vi "RFmx_An_IMD_Disp.vi"(6 "Target_Pwr(dBm)":dbl=1000000.0 format="%#_6p", 8 "Int_Bandwidth(Hz)":dbl=1000000.0 format="%#_6p", 9 "Signal_Bandwidth(Hz)":dbl=20000000.0 format="%#_6p", 10 "Tone_Spacing(Hz)":dbl=3000000.0 format="%#_6p", 11 "IMD_Spectrum_in":cluster{"x0":dbl, "dx":dbl, "y":sgl[]}={"x0"=989999984.4503028, "dx"=999.4019138756557, "y"=array[20012 elements]}) -> (2 "PeakPwrs_Data":sgl[](array[numeric])=[750000.0, -20.734814, 53.66733, 3.5194657] format="%#_6p", 3 "IMD_Spectrum_Out":cluster{"x0":dbl, "dx":dbl, "y":sgl[]}[](array[cluster])=[{"x0"=989999984.4503028, "dx"=999.4019138756557, "y"=array[20012 elements]}, {"x0"=989999984.4503028, "dx"=999.4019138756557, "y"=array[20012 elements]}])   [LabVIEW 2014]
panel:
  out "IMD_Spectrum":cluster{"x0":dbl, "dx":dbl, "y":sgl[]}[](graph)
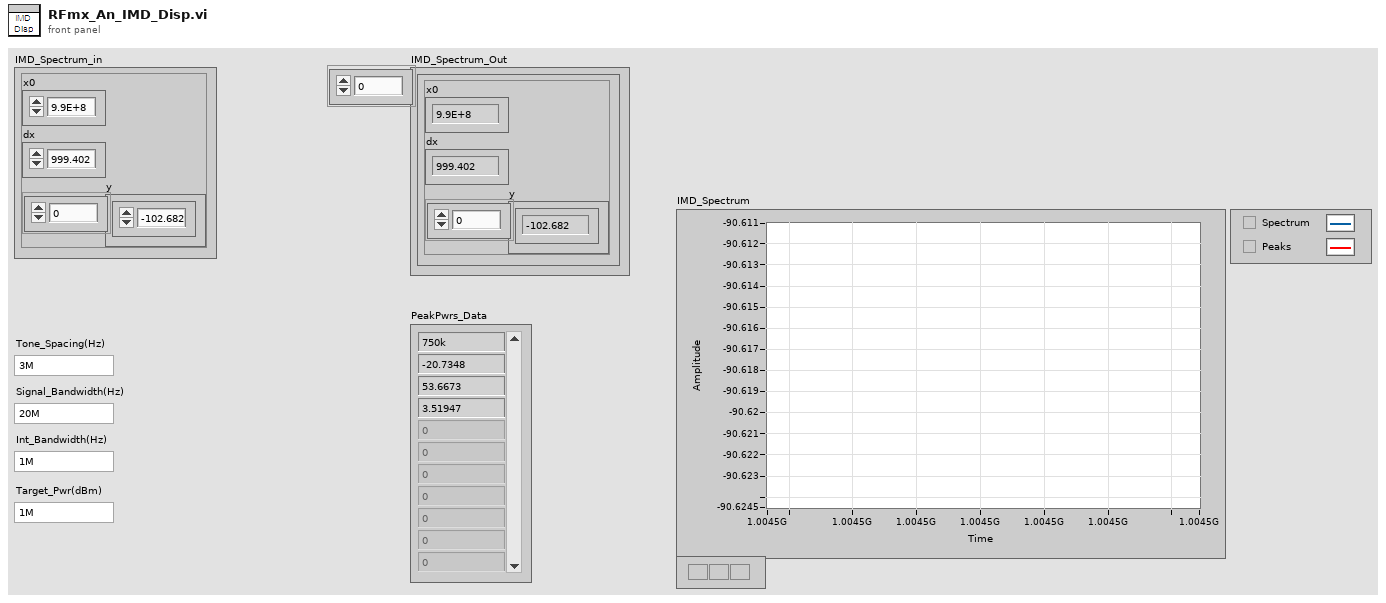
[diagram p1: front panel]
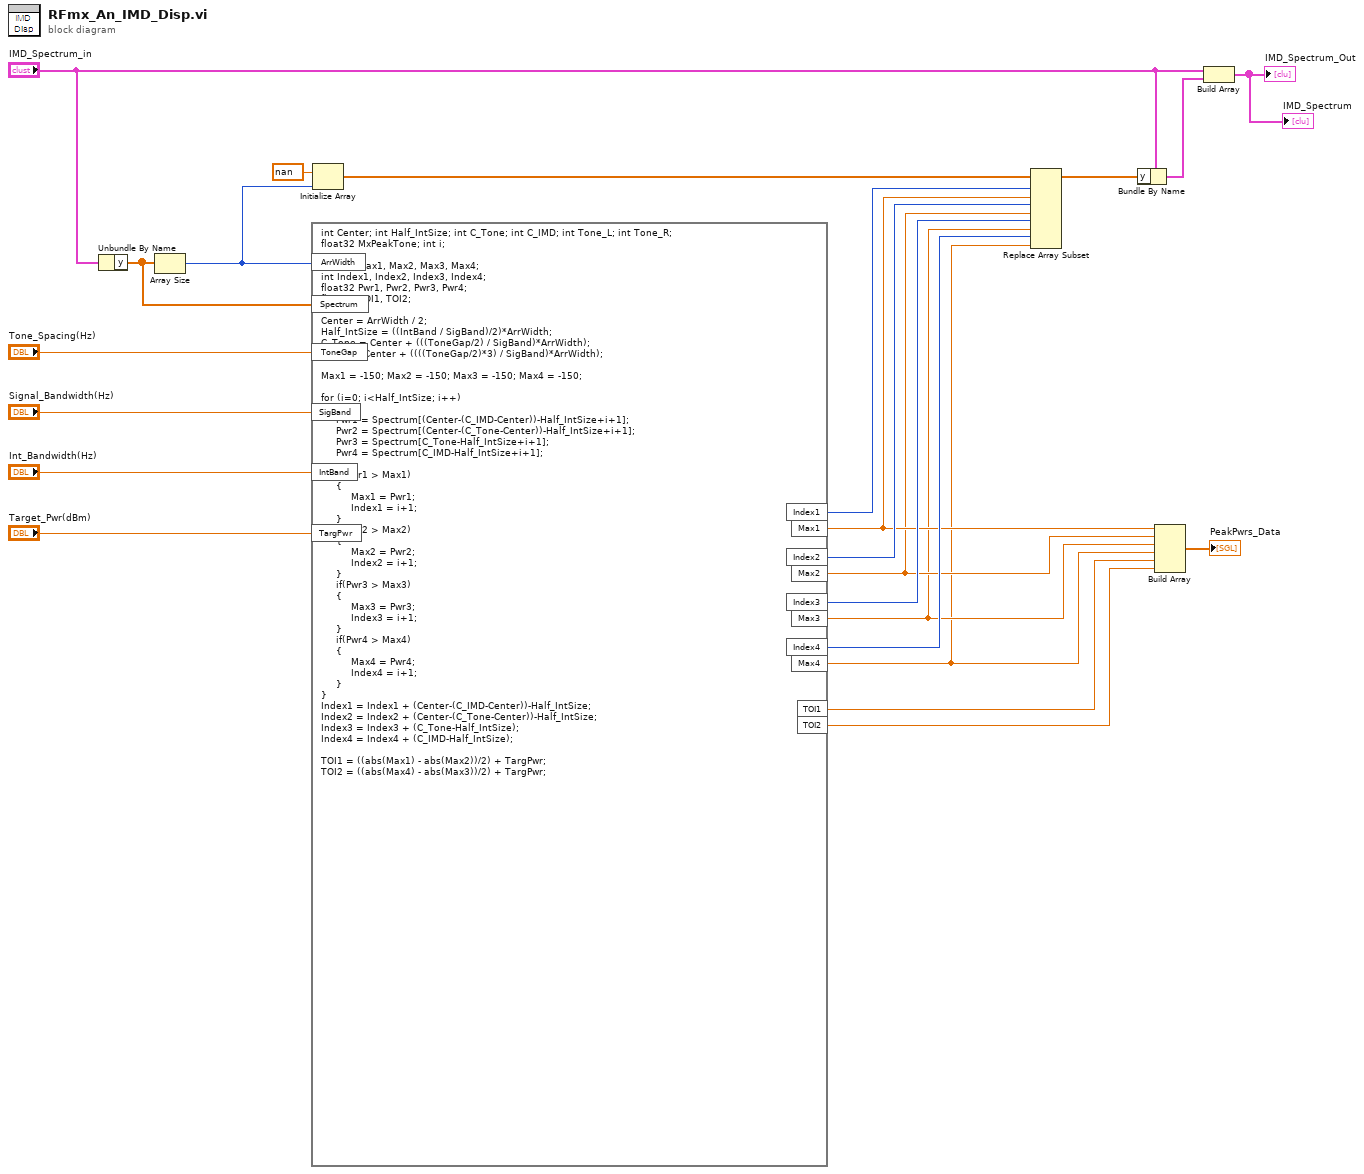
[diagram p0: block diagram]
diagram:
  n1 = Unbundle By Name("IMD_Spectrum_in") -> ("y"=w15:sgl[])
  n2 = Array Size(array=w15) -> (size(s)=w20:i32)
  n3 = formula code="int Center; int Half_IntSize; int C_Tone; int C_IMD; int Tone_L; int Tone_R;\nfloat32 MxPeakTone; int i;\n\nfloat32 Max1, Max2, Max3, Max4;\nint Index1, Index2, Index3, Index4;\nfloat32 Pwr1, Pwr2, Pwr3, Pwr4;\nfloat32 TOI1, TOI2;\n\nCenter = ArrWidth / 2;\nHalf_IntSize = ((IntBand / SigBand)/2)*ArrWidth;\nC_Tone = Center + (((ToneGap/2) / SigBand)*ArrWidth);\nC_IMD = Center + ((((ToneGap/2)*3) / SigBand)*ArrWidth);\n\nMax1 = -150; Max2 = -150; Max3 = -150; Max4 = -150;\n\nfor (i=0; i<Half_IntSize; i++)\n{\n     Pwr1 = Spectrum[(Center-(C_IMD-Center))-Half_IntSize+i+1];\n     Pwr2 = Spectrum[(Center-(C_Tone-Center))-Half_IntSize+i+1];\n     Pwr3 = Spectrum[C_Tone-Half_IntSize+i+1];\n     Pwr4 = Spectrum[C_IMD-Half_IntSize+i+1];\n\n     if(Pwr1 > Max1)\n     {\n          Max1 = Pwr1;\n          Index1 = i+1;\n     }\n     if(Pwr2 > Max2)\n     {\n          Max2 = Pwr2;\n          Index2 = i+1;\n     }     \n     if(Pwr3 > Max3)\n     {\n          Max3 = Pwr3;\n          Index3 = i+1;\n     }\n     if(Pwr4 > Max4)\n     {\n          Max4 = Pwr4;\n          Index4 = i+1;\n     }\n}\nIndex1 = Index1 + (Center-(C_IMD-Center))-Half_IntSize;\nIndex2 = Index2 + (Center-(C_Tone-Center))-Half_IntSize;\nIndex3 = Index3 + (C_Tone-Half_IntSize);\nIndex4 = Index4 + (C_IMD-Half_IntSize);\n\nTOI1 = ((abs(Max1) - abs(Max2))/2) + TargPwr;\nTOI2 = ((abs(Max4) - abs(Max3))/2) + TargPwr;"("ToneGap"="Tone_Spacing(Hz)", "SigBand"="Signal_Bandwidth(Hz)", "IntBand"="Int_Bandwidth(Hz)", "ArrWidth"=w20, "Spectrum"=w15, "TargPwr"="Target_Pwr(dBm)") -> ("Max3"=w6:sgl, "Index3"=w12:i32, "Max4"=w5:sgl, "Index4"=w11:i32, "Max1"=w8:sgl, "Index1"=w14:i32, "Max2"=w7:sgl, "Index2"=w13:i32, "TOI1"=w3:sgl, "TOI2"=w2:sgl)
  n4 = Initialize Array(sgl nan ("element"), w20) -> (w18:sgl[])
  n5 = Replace Array Subset(array=w18, new element #1=w8, index #1=w14, new element #2=w7, index #2=w13, new element #3=w6, index #3=w12, new element #4=w5, index #4=w11) -> (w17:sgl[])
  n6 = Bundle By Name(cluster="IMD_Spectrum_in", "y"=w17) -> (w16:cluster{"x0":dbl, "dx":dbl, "y":sgl[]})
  n7 = Build Array(w8, w7, w6, w5, w3, w2) -> (→"PeakPwrs_Data":sgl[])
  n8 = Build Array("IMD_Spectrum_in", w16) -> (→"IMD_Spectrum_Out" →"IMD_Spectrum":cluster{"x0":dbl, "dx":dbl, "y":sgl[]}[])
